vi "LoadXmlString.vi"(8 "error in":errorcluster caption="错误输入（无错误）", 10 "XmlString":string, 11 "PanelRootNode 输入":refnum<class "PanelRootNode.lvclass"> caption="DNL_LabVIEW Object in") -> (0 "error out":errorcluster caption="错误输出", 3 "PanelRootNode 输出":refnum<class "PanelRootNode.lvclass"> caption="DNL_LabVIEW Object out")   [LabVIEW 2013, in "PanelRootNode.lvclass"]
uses:
  PanelRootNode.lvclass
  <vilib>/xml/Close Reference(Node).vi
  <vilib>/xml/NI_XML.lvlib
  <resource>/objmgr/DOMUserDefRef.rc
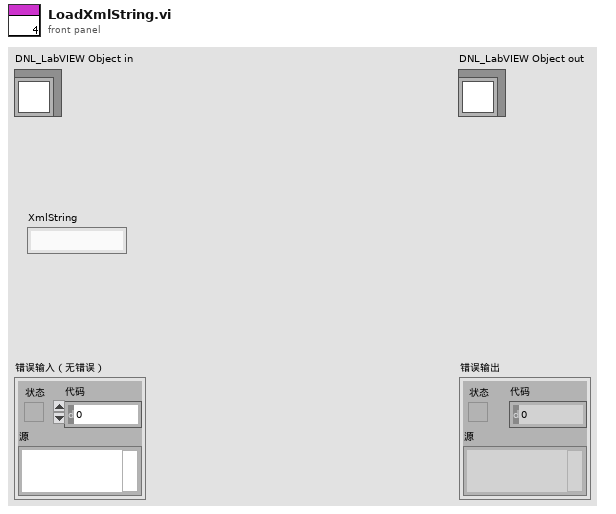
[diagram p1: front panel]
types:
  T1 = cluster{"DOM Ref":refnum<k20>, "Node Ref":refnum<k20>}
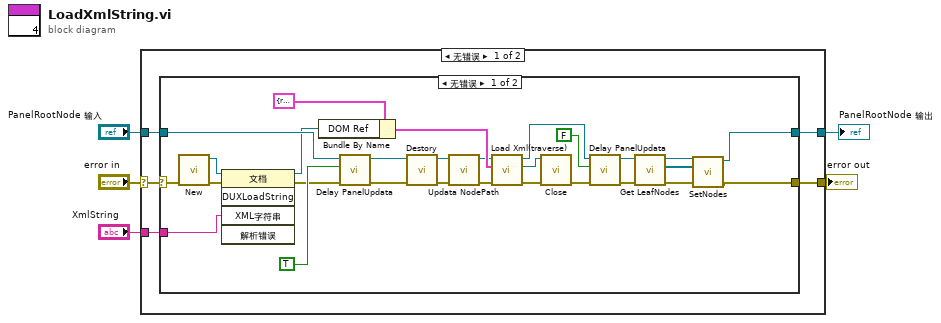
[diagram p0: block diagram]
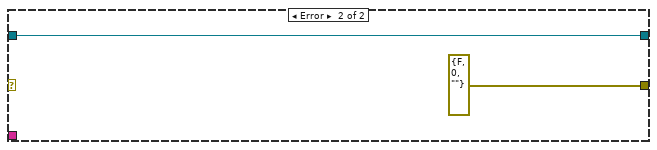
[diagram p2: hidden frame]
diagram:
  n1 = case shown="无错误" "error in" {
    selector: "error in" -> [w7 w42]
    tunnel: [w9 w42] -> w4
    tunnel: [w10 w41] -> w2
    tunnel: "PanelRootNode 输入" -> [w8 w41]
    tunnel: "XmlString" -> [w6 _]
    frame No Error {
      n2 = case shown="无错误" w7 {
        selector: w7 -> [w23 _]
        tunnel: w8 -> [w30 w40]
        tunnel: [w12 w40] -> w10
        tunnel: [w11 errorcluster {"status"=FALSE, "code"=0, "source"=""} ("error out")] -> w9
        tunnel: w6 -> [w18 _]
        frame No Error {
          n3 = call <vilib>:"New.vi"("error in (no error)"=w23) -> ("error out"=w20:errorcluster, "DOM document out"=w22:refnum<k20>)  [unwired: 7 in]
          n4 = invoke class="文档" method="DUXLoadString"(reference=w22, error in=w20, "XML字符串"=w18) -> (reference out=w21:refnum<k20>, error out=w19:errorcluster)  [unwired: 2 in, 3 out]
          n5 = Bundle By Name(cluster=T1 {"DOM Ref"=refnum, "Node Ref"=refnum} ("Data in"), "DOM Ref"=w21) -> (w36:T1)
          n6 = call "Delay PanelUpdata.vi"("error in (no error)"=w19, "延迟前面板更新"=TRUE, "PanelRootNode 输入"=w30) -> ("error out"=w28:errorcluster, "PanelRootNode 输出"=w29:refnum<class "PanelRootNode.lvclass">)  [unwired: 7 in]
          n7 = call-dynamic "Destory.vi"("error in (no error)"=w28, "PanelRootNode 输入"=w29) -> ("error out"=w32:errorcluster, "PanelRootNode 输出"=w34:refnum<class "PanelRootNode.lvclass">)  [unwired: 8 in]
          n8 = call-dynamic "Updata NodePath.vi"("error in"=w32, "PanelLinkNode 输入"=w34) -> ("error out"=w31:errorcluster, "PanelLinkNode 输出"=w33:refnum<class "PanelRootNode.lvclass">)  [unwired: 8 in]
          n9 = call "Load Xml(traverse).vi"("error in"=w31, "Data in"=w36, "PanelRootNode.lvclass"=w33) -> ("error out"=w35:errorcluster, "DOM Ref"=w38:refnum<k20>, "PanelRootNode out"=w26:refnum<class "PanelRootNode.lvclass">)  [unwired: 6 in]
          n10 = call-poly <vilib>:"Close.vi"("error in (no error)"=w35, "node"=w38) -> ("error out"=w24:errorcluster)  [unwired: 7 in]
          n11 = call "Delay PanelUpdata.vi"("error in (no error)"=w24, "延迟前面板更新"=FALSE, "PanelRootNode 输入"=w26) -> ("error out"=w16:errorcluster, "PanelRootNode 输出"=w17:refnum<class "PanelRootNode.lvclass">)  [unwired: 7 in]
          n12 = call-dynamic "Get LeafNodes.vi"("error in (no error)"=w16, "PanelRootNode 输入"=w17) -> ("error out"=w13:errorcluster, "DataNode[]"=w15:refnum<data-value>[], "PanelRootNode 输出"=w14:refnum<class "PanelRootNode.lvclass">)  [unwired: 7 in]
          n13 = call "SetNodes.vi"("error in (no error)"=w13, "LeafNodes[]"=w15, "PanelRootNode 输入"=w14) -> ("error out"=w11:errorcluster, "PanelRootNode 输出"=w12:refnum<class "PanelRootNode.lvclass">)  [unwired: 7 in]
        }
        frame Error {
        }
      }
    }
    frame Error {
    }
  }
  "error out" <- w4
  "PanelRootNode 输出" <- w2
